vi "Versioned Load.vi"(10 "path":path) -> (0 "Reversals":T10, 1 "Trajectory Data":T1, 2 "Zero V":bool, 3 "Commands out":cluster{"Time (s)":dbl, T8, bool}[](array[cluster]), 4 "Fields":T7 {"Overrides"."Angle Override" step=5.0; "Overrides"."Velocity Override" step=5.0; "Overrides"."Angular Override" step=5.0; "Angular Limits"."Jerk (deg/s^3)" min=0.0 step=1.0; "Angular Limits"."Accel (deg/s^2)" min=0.0; "Angular Limits"."Velocity (deg/s)" min=0.0}, 5 "Points out":cluster{"x":dbl, "y":dbl, "th":dbl}[](array[cluster]), 6 "Trajectory Meta":cluster{"Drive Type":T3, "Path Type":T4}, 7 "Overall":cluster{"Time (s)":dbl, "Distance (ft)":dbl})   [LabVIEW 2025]
uses:
  Types/Single Cmd Info.ctl
  <vilib>/picture/picture.llb/imagedata.ctl
  Types/Overrides.ctl
  Types/Angluar Limits.ctl
  Types/Drive Type.ctl
  Types/Path Type.ctl
  Types/Trajectory Data.ctl
  Types/Segment Type.ctl
  Types/Availible Command systems for auto.ctl
  Types/Limits.ctl
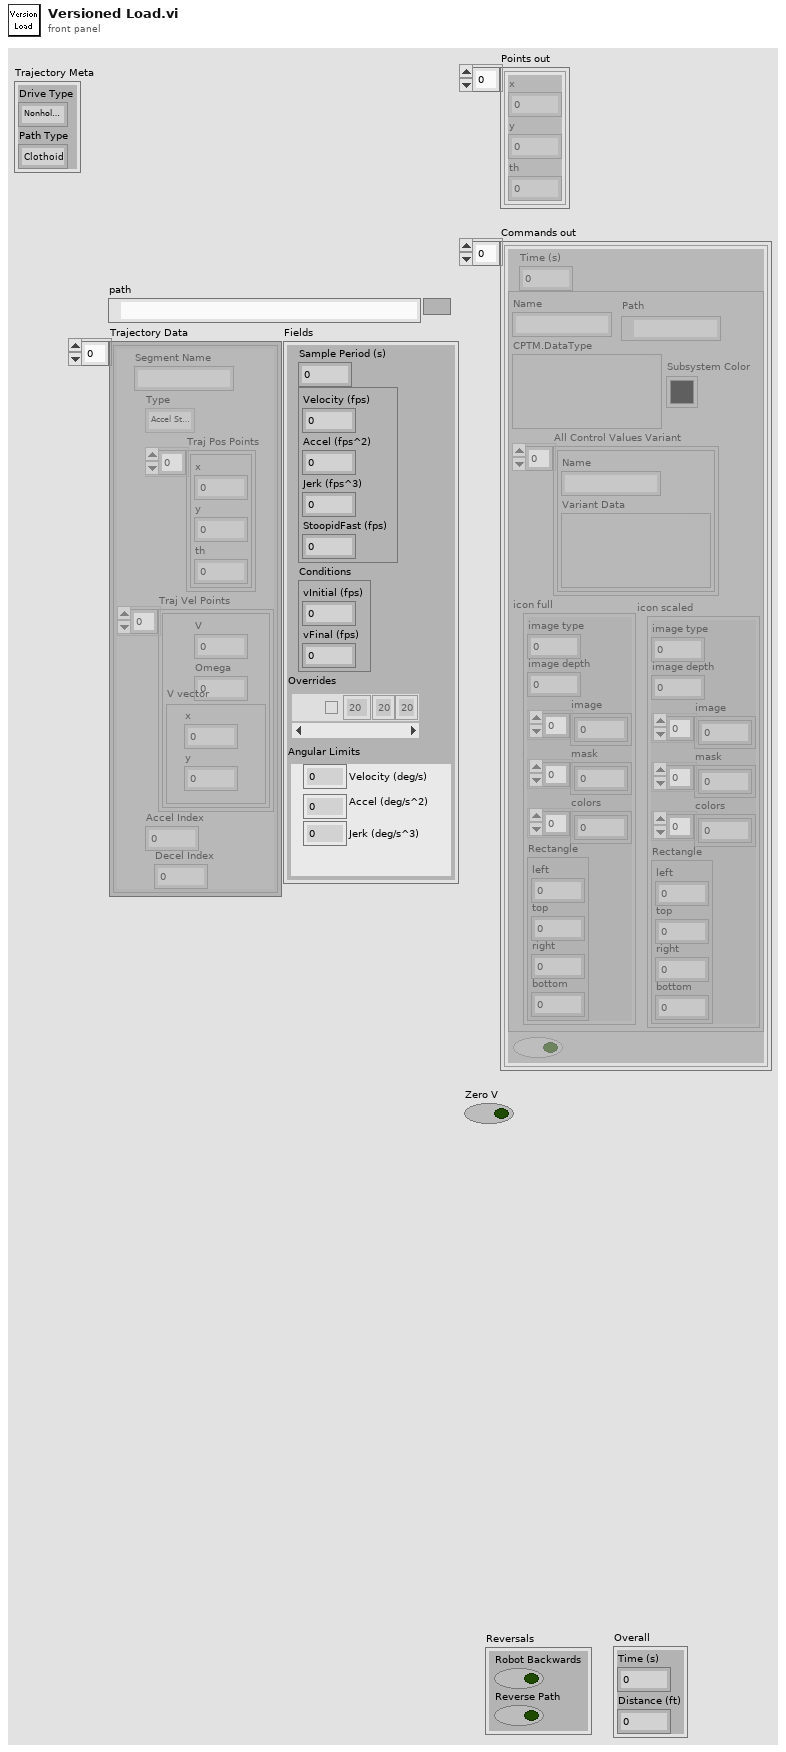
[diagram p1: front panel]
types:
  T1 = typedef "Trajectory Data.ctl" = cluster{"Segment Name":string, "Type":T2, "Traj Pos Points":cluster{"x":dbl, "y":dbl, "th":dbl}[], "Traj Vel Points":cluster{"V":dbl, "Omega":dbl, "V vector":cluster{"y":dbl, "x":dbl}}[], "Accel Index":i32, "Decel Index":i32}[]
  T2 = typedef "Segment Type.ctl" = enum16{"Accel Straight", "Const Straight", "Blend", "Circle", "Bezier"}
  T3 = typedef "Drive Type.ctl" = enum16{"Nonholonomic", "Holonomic"}
  T4 = typedef "Path Type.ctl" = enum16{"Clothoid", "Bezier"}
  T5 = typedef "Overrides.ctl" = cluster{"Count":string, "Angular Override":dbl, "Enabled?":bool, "Velocity Override":dbl, "Angle Override":dbl}[]
  T6 = typedef "Angluar Limits.ctl" = cluster{"Velocity (deg/s)":dbl, "Accel (deg/s^2)":dbl, "Jerk (deg/s^3)":dbl}
  T7 = cluster{"Sample Period (s)":dbl, cluster{"Velocity (fps)":dbl, "Accel (fps^2)":dbl, "Jerk (fps^3)":dbl, "StoopidFast (fps)":dbl}, "Conditions":cluster{"vInitial (fps)":dbl, "vFinal (fps)":dbl}, "Overrides":T5, "Angular Limits":T6}
  T8 = typedef "Single Cmd Info.ctl" = cluster{"Name":string, "CPTM.DataType":variant, "All Control Values Variant":cluster{"Name":string, "Variant Data":variant}[], "icon full":T9, "icon scaled":T9, "Path":path, "Subsystem Color":u32}
  T9 = typedef "imagedata.ctl" = cluster{"image type":i32, "image depth":i32, "image":u8[], "mask":u8[], "colors":u32[], "Rectangle":cluster{"left":i16, "top":i16, "right":i16, "bottom":i16}}
  T10 = cluster{"Robot Backwards":bool, "Reverse Path":bool}
  T11 = cluster{"Segment Name":string, "Type":T2, "Traj Pos Points":cluster{"x":dbl, "y":dbl, "th":dbl}[], "Traj Vel Points":cluster{"V":dbl, "Omega":dbl}[], "Accel Index":i32, "Decel Index":i32}[]
  T12 = cluster{"Sample Period (s)":dbl, "Limits 2":cluster{"Velocity (fps)":dbl, "Acceleration (fps^2)":dbl, "Jerk (fps^3)":dbl}, "Conditions":cluster{"vInitial (fps)":dbl, "vFinal (fps)":dbl}, " Acceleration Overrides":cluster{"Angular \nAccelerations":dbl[], "Accel Override Bools":bool[]}}
  T13 = cluster{"Velocity":dbl, "Sample Time":dbl, "Accel":dbl}
  T14 = cluster{"Sample Period (s)":dbl, "Limits":cluster{"Velocity (fps)":dbl, "Acceleration (fps^2)":dbl, "Jerk (fps^3)":dbl}, "Conditions":cluster{"vInitial (fps)":dbl, "vFinal (fps)":dbl}}
  T15 = cluster{"Sample Period (s)":dbl, "Limits":cluster{"Velocity (fps)":dbl, "Acceleration (fps^2)":dbl, "Jerk (fps^3)":dbl}, "Conditions":cluster{"vInitial (fps)":dbl, "vFinal (fps)":dbl}, "Min Rads":dbl[]}
  T16 = typedef "Availible Command systems for auto.ctl" = u16
  T17 = cluster{"Time into Path":dbl, "System":T16, "Item Selected?":bool, "System Selection":T16}[]
  T18 = cluster{"Sample Period (s)":dbl, "Limits 2":cluster{"Velocity (fps)":dbl, "Acceleration (fps^2)":dbl, "Jerk (fps^3)":dbl, "Stoopid Fast":dbl}, "Conditions":cluster{"vInitial (fps)":dbl, "vFinal (fps)":dbl}, " Acceleration Overrides":cluster{"Angular \nAccelerations":dbl[], "Accel Override Bools":bool[]}}
  T19 = cluster{"Sample Period (s)":dbl, "Limits":cluster{"Velocity (fps)":dbl, "Accel (fps^2)":dbl, "Turn Accel (fps^2)":dbl, "Jerk (fps^3)":dbl}, "Conditions":cluster{"vInitial (fps)":dbl, "vFinal (fps)":dbl}, cluster{dbl[], bool[]}}
  T20 = cluster{"Reverse Path":bool, "Robot Backwards":bool}
  T21 = typedef "Limits.ctl" = cluster{"Velocity (fps)":dbl, "Accel (fps^2)":dbl, "Jerk (fps^3)":dbl, "StoopidFast (fps)":dbl}
  T22 = cluster{"Sample Period (s)":dbl, "Limits":T21, "Conditions":cluster{"vInitial (fps)":dbl, "vFinal (fps)":dbl}, "Overrides":T5, "Angular Limits":T6}
  T23 = cluster{"Velocity":dbl, "Accel":dbl, "Accel":dbl, "Velocity":dbl}
  T24 = cluster{"Velocity (fps)":dbl, "Acceleration (fps^2)":dbl, "Jerk (fps^3)":dbl}
  T25 = cluster{"vInitial (fps)":dbl, "vFinal (fps)":dbl}
  T26 = cluster{"Velocity (fps)":dbl, "Acceleration (fps^2)":dbl, "Jerk (fps^3)":dbl, "Velocity (fps)":dbl}
  T27 = cluster{string, "Angular Multiplier":dbl, bool, "Velocity (fps)":dbl, "Velocity (fps)":dbl}
  T28 = cluster{"Angular \nAccelerations":dbl[], "Accel Override Bools":bool[]}
  T29 = cluster{"Velocity (fps)":dbl, "Acceleration (fps^2)":dbl, "Jerk (fps^3)":dbl, "Stoopid Fast":dbl}
  T30 = cluster{"Velocity (fps)":dbl, "Accel (fps^2)":dbl, "Turn Accel (fps^2)":dbl, "Jerk (fps^3)":dbl}
  T31 = cluster{"Velocity (fps)":dbl, "Accel (fps^2)":dbl, "Jerk (fps^3)":dbl, "StoopidFast (fps)":dbl}
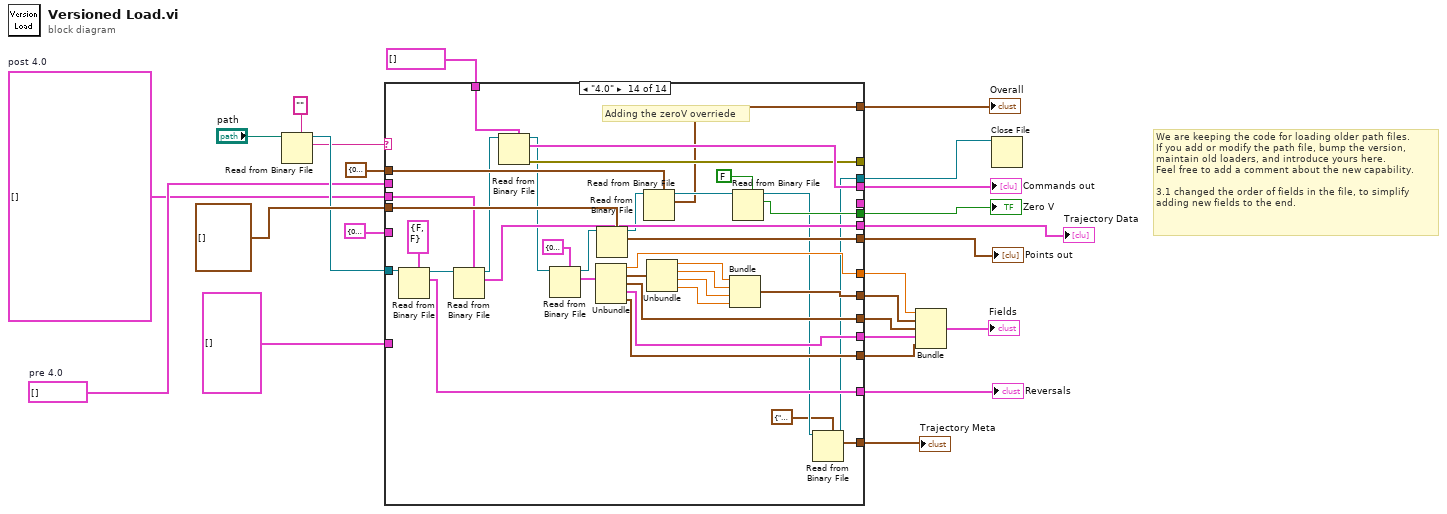
[diagram p0: block diagram]
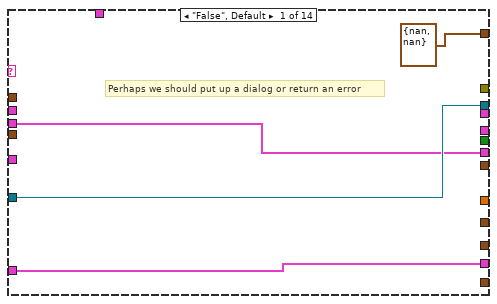
[diagram p2: hidden frame]
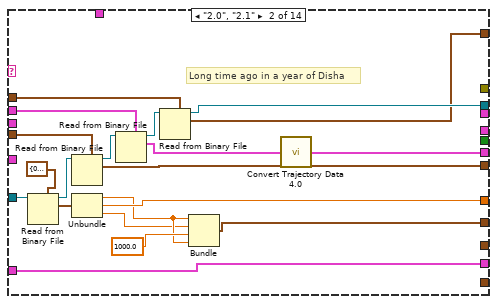
[diagram p3: hidden frame]
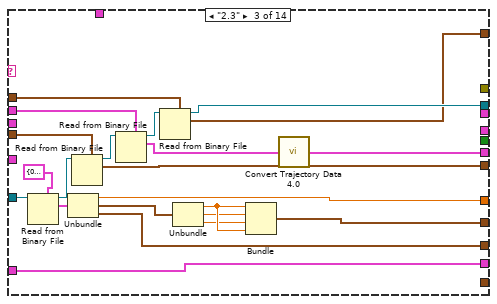
[diagram p4: hidden frame]
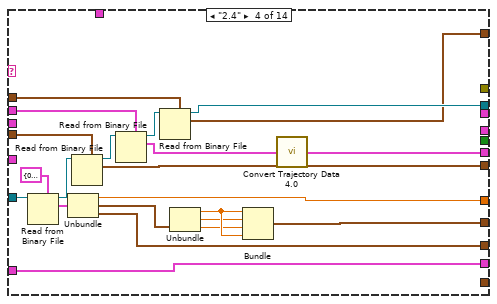
[diagram p5: hidden frame]
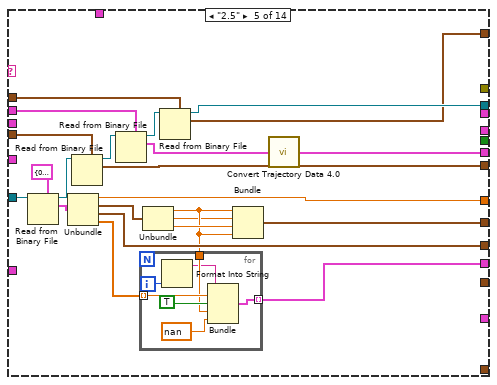
[diagram p6: hidden frame]
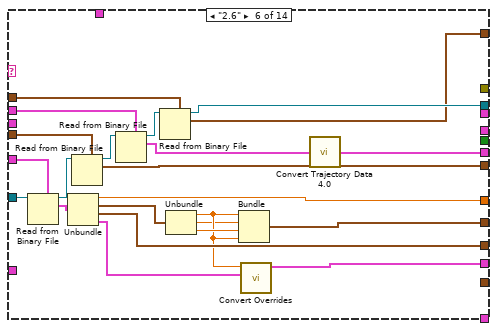
[diagram p7: hidden frame]
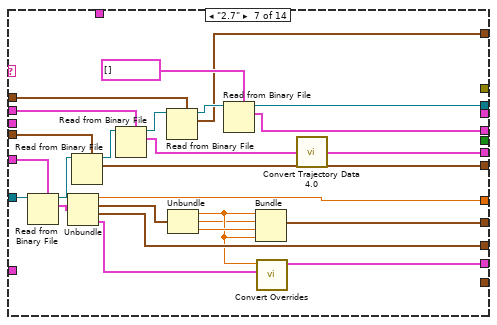
[diagram p8: hidden frame]
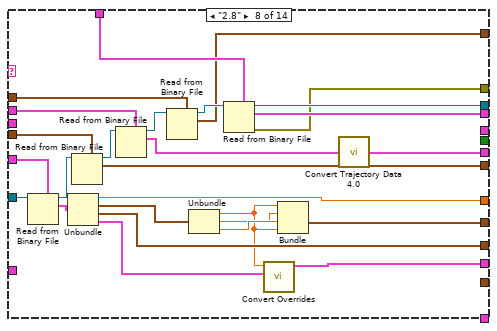
[diagram p9: hidden frame]
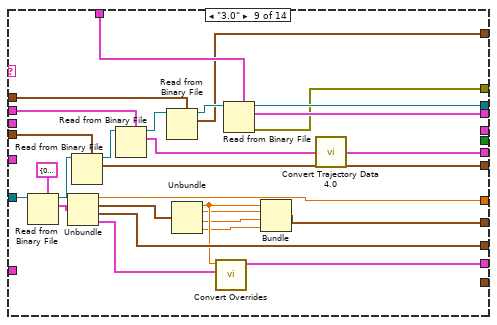
[diagram p10: hidden frame]
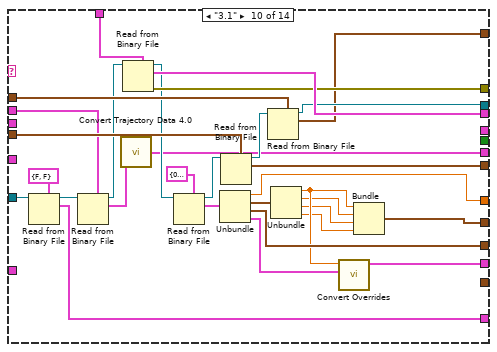
[diagram p11: hidden frame]
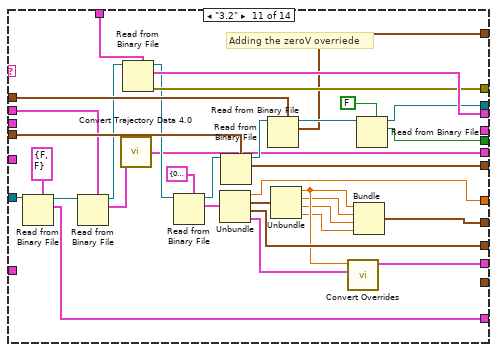
[diagram p12: hidden frame]
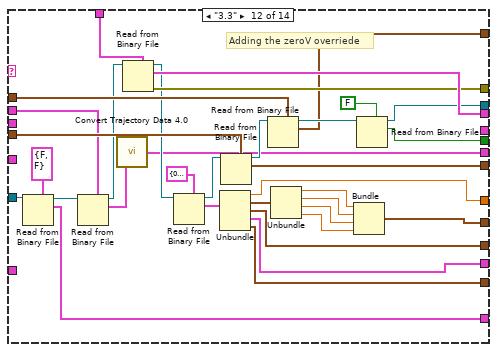
[diagram p13: hidden frame]
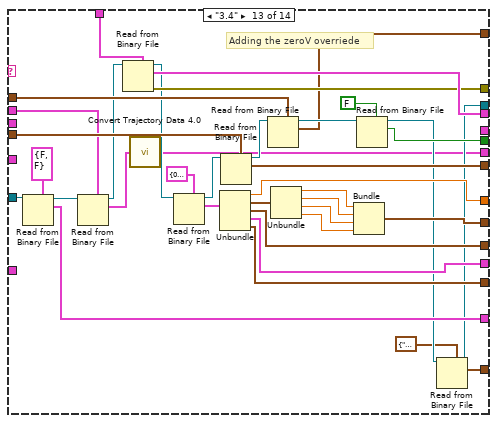
[diagram p14: hidden frame]
diagram:
  w3 = T11 []  # pre 4.0
  w2 = T1 []  # post 4.0
  # "We are keeping the code for loading older path files.\nIf you add or modify the path file, bump the version,\nmaintain old loaders, and introduce yours here.\nFeel free to add a comment about the new capability.\n\n3.1 changed the order of fields in the file, to simplify\nadding new fields to the end."
  n1 = Read from Binary File(5:"" ("String"), 11:"path") -> (2:w9:string, 3:w10:refnum<file>)  [unwired: 4 in, 2 out]
  n2 = case shown="\"4.0\"" w9 {
    tunnel: w10 -> [w29 w48 w70 w92 w115 w145 w171 w198 w226 w247 w281 w315 w352 w389]
    tunnel: cluster{"x":dbl, "y":dbl, "th":dbl}[] [] ("Points in") -> [_ w46 w68 w90 w113 w143 w169 w196 w224 w256 w290 w324 w361 w397]
    tunnel: [_ w45 w67 w89 w112 w142 w168 w195 w223 w255 w289 w323 w360 w396] -> w15
    tunnel: w3 -> [_ w44 w66 w88 w111 w141 w167 w194 w222 w254 w288 w322 w359 _]
    tunnel: cluster{"Time (s)":dbl, "Distance (ft)":dbl} {"Time (s)"=0.0, "Distance (ft)"=0.0} ("Cluster 4") -> [_ w42 w64 w86 w109 w139 w165 w192 w220 w253 w287 w321 w358 w395]
    tunnel: [w29 w40 w62 w84 w107 w137 w159 w186 w214 w243 w263 w300 w329 w366] -> w12
    tunnel: [_ w38 w61 w83 w106 w136 w163 w190 w218 w230 w265 w302 w339 w376] -> w22
    tunnel: [_ w34 w55 w76 w100 w131 w153 w181 w202 w235 w270 w307 w344 w381] -> w23
    tunnel: [_ _ w60 w82 w105 w135 w162 w189 w217 w252 w286 w320 w357 w394] -> w24
    tunnel: [w28 w33 w54 w75 w99 w129 w150 w178 w208 w239 w274 w295 w333 w370] -> w25
    tunnel: [w26 w30 w50 w72 w94 w124 w147 w173 w200 w228 w259 w293 w327 w393] -> w1
    tunnel: [_ _ _ _ _ _ w158 _ _ _ _ _ _ _] -> _
    tunnel: cluster{"Time (s)":dbl, T8, bool}[] [] ("Commands in") -> [_ _ _ _ _ _ _ w185 w213 w250 w284 w318 w355 w392]
    tunnel: [_ _ _ _ _ _ _ w184 w212 w249 w283 w317 w354 w391] -> w17
    tunnel: [_ _ _ _ _ _ _ w183 w211 w248 w282 w316 w353 w390] -> _
    tunnel: T12 {"Sample Period (s)"=0.0, "Limits 2"={"Velocity (fps)"=0.0, "Acceleration (fps^2)"=0.0, "Jerk (fps^3)"=0.0}, "Conditions"={"vInitial (fps)"=0.0, "vFinal (fps)"=0.0}, " Acceleration Overrides"={"Angular \nAccelerations"=[], "Accel Override Bools"=[]}} ("Cluster") -> [_ _ _ _ _ w133 w156 w179 _ _ _ _ _ _]
    tunnel: [_ _ _ _ _ _ _ _ _ w238 w273 w309 w346 w383] -> w19
    tunnel: T5 [] ("Overrides") -> [w28 w33 w54 w75 _ _ _ _ _ _ _ _ _ _]
    tunnel: [_ _ _ _ _ _ _ _ _ _ w261 w298 w336 w373] -> w20
    tunnel: [cluster{"Time (s)":dbl, "Distance (ft)":dbl} {"Time (s)"=nan, "Distance (ft)"=nan} ("Cluster 4") w31 w51 w73 w95 w125 w148 w174 w201 w229 w260 w297 w335 w372] -> w7
    tunnel: [_ _ _ _ _ _ _ _ _ _ _ w294 w332 w369] -> w5
    tunnel: [_ _ _ _ _ _ _ _ _ _ _ _ w328 w365] -> w4
    tunnel: w2 -> [w26 _ _ _ _ _ _ _ _ _ _ _ _ w364]
    frame "False", Default {
      # "Perhaps we should put up a dialog or return an error"
    }
    frame "2.0", "2.1" {
      # "Long time ago in a year of Disha"
      n3 = Read from Binary File(5:T13 {"Velocity"=0.0, "Sample Time"=0.0, "Accel"=0.0}, 11:w48) -> (2:w49:T13, 3:w47:refnum<file>)  [unwired: 4 in, 2 out]
      n4 = Read from Binary File(5:w46, 11:w47) -> (2:w45:cluster{"x":dbl, "y":dbl, "th":dbl}[], 3:w43:refnum<file>)  [unwired: 4 in, 2 out]
      n5 = Unbundle(w49) -> ("Velocity"=w35:dbl, "Sample Time"=w38:dbl, "Accel"=w32:dbl)
      n6 = Read from Binary File(5:w44, 11:w43) -> (2:w36:T11, 3:w41:refnum<file>)  [unwired: 4 in, 2 out]
      n7 = Read from Binary File(5:w42, 11:w41) -> (2:w31:cluster{"Time (s)":dbl, "Distance (ft)":dbl}, 3:w40:refnum<file>)  [unwired: 4 in, 2 out]
      n8 = Bundle("Velocity"=w35, "Accel"=w32, "Accel"=1000.0, "Velocity"=w35) -> (w34:T23)  [unwired: 1 in]
      n9 = call "Convert Trajectory Data 4.0.vi"("pre 4.0"=w36) -> ("post 4.0"=w30:T1)
    }
    frame "2.3" {
      n10 = Read from Binary File(5:T14 {"Sample Period (s)"=0.0, "Limits"={"Velocity (fps)"=0.0, "Acceleration (fps^2)"=0.0, "Jerk (fps^3)"=0.0}, "Conditions"={"vInitial (fps)"=0.0, "vFinal (fps)"=0.0}}, 11:w70) -> (2:w71:T14, 3:w69:refnum<file>)  [unwired: 4 in, 2 out]
      n11 = Unbundle(w71) -> ("Sample Period (s)"=w61:dbl, "Limits"=w52:T24, "Conditions"=w60:T25)
      n12 = Read from Binary File(5:w68, 11:w69) -> (2:w67:cluster{"x":dbl, "y":dbl, "th":dbl}[], 3:w65:refnum<file>)  [unwired: 4 in, 2 out]
      n13 = Read from Binary File(5:w66, 11:w65) -> (2:w58:T11, 3:w63:refnum<file>)  [unwired: 4 in, 2 out]
      n14 = Read from Binary File(5:w64, 11:w63) -> (2:w51:cluster{"Time (s)":dbl, "Distance (ft)":dbl}, 3:w62:refnum<file>)  [unwired: 4 in, 2 out]
      n15 = Unbundle(w52) -> ("Velocity (fps)"=w57:dbl, "Acceleration (fps^2)"=w53:dbl, "Jerk (fps^3)"=w56:dbl)
      n16 = Bundle("Velocity (fps)"=w57, "Acceleration (fps^2)"=w53, "Jerk (fps^3)"=w56, "Velocity (fps)"=w57) -> (w55:T26)  [unwired: 1 in]
      n17 = call "Convert Trajectory Data 4.0.vi"("pre 4.0"=w58) -> ("post 4.0"=w50:T1)
    }
    frame "2.4" {
      n18 = Read from Binary File(5:T14 {"Sample Period (s)"=0.0, "Limits"={"Velocity (fps)"=0.0, "Acceleration (fps^2)"=0.0, "Jerk (fps^3)"=0.0}, "Conditions"={"vInitial (fps)"=0.0, "vFinal (fps)"=0.0}}, 11:w92) -> (2:w93:T14, 3:w91:refnum<file>)  [unwired: 4 in, 2 out]
      n19 = Unbundle(w93) -> ("Sample Period (s)"=w83:dbl, "Limits"=w77:T24, "Conditions"=w82:T25)
      n20 = Read from Binary File(5:w90, 11:w91) -> (2:w89:cluster{"x":dbl, "y":dbl, "th":dbl}[], 3:w87:refnum<file>)  [unwired: 4 in, 2 out]
      n21 = Read from Binary File(5:w88, 11:w87) -> (2:w80:T11, 3:w85:refnum<file>)  [unwired: 4 in, 2 out]
      n22 = Read from Binary File(5:w86, 11:w85) -> (2:w73:cluster{"Time (s)":dbl, "Distance (ft)":dbl}, 3:w84:refnum<file>)  [unwired: 4 in, 2 out]
      n23 = Unbundle(w77) -> ("Velocity (fps)"=w79:dbl, "Acceleration (fps^2)"=w74:dbl, "Jerk (fps^3)"=w78:dbl)
      n24 = Bundle("Velocity (fps)"=w79, "Acceleration (fps^2)"=w74, "Jerk (fps^3)"=w78, "Velocity (fps)"=w79) -> (w76:T26)  [unwired: 1 in]
      n25 = call "Convert Trajectory Data 4.0.vi"("pre 4.0"=w80) -> ("post 4.0"=w72:T1)
    }
    frame "2.5" {
      n26 = Read from Binary File(5:T15 {"Sample Period (s)"=0.0, "Limits"={"Velocity (fps)"=0.0, "Acceleration (fps^2)"=0.0, "Jerk (fps^3)"=0.0}, "Conditions"={"vInitial (fps)"=0.0, "vFinal (fps)"=0.0}, "Min Rads"=[20.0, 20.0, 20.0, 20.0, 20.0]}, 11:w115) -> (2:w116:T15, 3:w114:refnum<file>)  [unwired: 4 in, 2 out]
      n27 = Unbundle(w116) -> ("Sample Period (s)"=w106:dbl, "Limits"=w101:T24, "Conditions"=w105:T25, "Min Rads"=w98:dbl[])
      n28 = Read from Binary File(5:w113, 11:w114) -> (2:w112:cluster{"x":dbl, "y":dbl, "th":dbl}[], 3:w110:refnum<file>)  [unwired: 4 in, 2 out]
      n29 = Read from Binary File(5:w111, 11:w110) -> (2:w103:T11, 3:w108:refnum<file>)  [unwired: 4 in, 2 out]
      n30 = Unbundle(w101) -> ("Velocity (fps)"=w97:dbl, "Acceleration (fps^2)"=w96:dbl, "Jerk (fps^3)"=w102:dbl)
      n31 = for {
        tunnel: [w122] -> w99 mode=indexing
        tunnel: w98 -> [w121] mode=indexing
        tunnel: w97 -> [w120]
        i -> [w119]
        n32 = Format Into String(w119) -> (resulting string=w118:string)  [unwired: 3 in, 1 out]
        n33 = Bundle(w118, "Angular Multiplier"=w121, TRUE, "Velocity (fps)"=w120, "Velocity (fps)"=nan) -> (w122:T27)  [unwired: 1 in]
      }
      n34 = Read from Binary File(5:w109, 11:w108) -> (2:w95:cluster{"Time (s)":dbl, "Distance (ft)":dbl}, 3:w107:refnum<file>)  [unwired: 4 in, 2 out]
      n35 = Bundle("Velocity (fps)"=w97, "Acceleration (fps^2)"=w96, "Jerk (fps^3)"=w102, "Velocity (fps)"=w97) -> (w100:T26)  [unwired: 1 in]
      n36 = call "Convert Trajectory Data 4.0.vi"("pre 4.0"=w103) -> ("post 4.0"=w94:T1)
    }
    frame "2.6" {
      n37 = Read from Binary File(5:w133, 11:w145) -> (2:w146:T12, 3:w144:refnum<file>)  [unwired: 4 in, 2 out]
      n38 = Unbundle(w146) -> ("Sample Period (s)"=w136:dbl, "Limits 2"=w130:T24, "Conditions"=w135:T25, "Acceleration Overrides"=w127:T28)
      n39 = Read from Binary File(5:w143, 11:w144) -> (2:w142:cluster{"x":dbl, "y":dbl, "th":dbl}[], 3:w140:refnum<file>)  [unwired: 4 in, 2 out]
      n40 = Read from Binary File(5:w141, 11:w140) -> (2:w134:T11, 3:w138:refnum<file>)  [unwired: 4 in, 2 out]
      n41 = Read from Binary File(5:w139, 11:w138) -> (2:w125:cluster{"Time (s)":dbl, "Distance (ft)":dbl}, 3:w137:refnum<file>)  [unwired: 4 in, 2 out]
      n42 = Unbundle(w130) -> ("Velocity (fps)"=w128:dbl, "Acceleration (fps^2)"=w126:dbl, "Jerk (fps^3)"=w132:dbl)
      n43 = Bundle("Velocity (fps)"=w128, "Acceleration (fps^2)"=w126, "Jerk (fps^3)"=w132, "Velocity (fps)"=w128) -> (w131:T26)  [unwired: 1 in]
      n44 = call "Convert Overrides.vi"("Cluster"=w127, "Velocity (fps)"=w128) -> ("Overrides"=w129:T5)  [unwired: 9 in]
      n45 = call "Convert Trajectory Data 4.0.vi"("pre 4.0"=w134) -> ("post 4.0"=w124:T1)
    }
    frame "2.7" {
      n46 = Read from Binary File(5:w156, 11:w171) -> (2:w172:T12, 3:w170:refnum<file>)  [unwired: 4 in, 2 out]
      n47 = Unbundle(w172) -> ("Sample Period (s)"=w163:dbl, "Limits 2"=w154:T24, "Conditions"=w162:T25, "Acceleration Overrides"=w151:T28)
      n48 = Read from Binary File(5:w169, 11:w170) -> (2:w168:cluster{"x":dbl, "y":dbl, "th":dbl}[], 3:w166:refnum<file>)  [unwired: 4 in, 2 out]
      n49 = Read from Binary File(5:w167, 11:w166) -> (2:w161:T11, 3:w164:refnum<file>)  [unwired: 4 in, 2 out]
      n50 = Read from Binary File(5:w165, 11:w164) -> (2:w148:cluster{"Time (s)":dbl, "Distance (ft)":dbl}, 3:w160:refnum<file>)  [unwired: 4 in, 2 out]
      n51 = Unbundle(w154) -> ("Velocity (fps)"=w152:dbl, "Acceleration (fps^2)"=w149:dbl, "Jerk (fps^3)"=w155:dbl)
      n52 = Read from Binary File(5:T17 [] ("Commands"), 11:w160) -> (2:w158:T17, 3:w159:refnum<file>)  [unwired: 4 in, 2 out]
      n53 = Bundle("Velocity (fps)"=w152, "Acceleration (fps^2)"=w149, "Jerk (fps^3)"=w155, "Velocity (fps)"=w152) -> (w153:T26)  [unwired: 1 in]
      n54 = call "Convert Overrides.vi"("Cluster"=w151, "Velocity (fps)"=w152) -> ("Overrides"=w150:T5)  [unwired: 9 in]
      n55 = call "Convert Trajectory Data 4.0.vi"("pre 4.0"=w161) -> ("post 4.0"=w147:T1)
    }
    frame "2.8" {
      n56 = Read from Binary File(5:w179, 11:w198) -> (2:w199:T12, 3:w197:refnum<file>)  [unwired: 4 in, 2 out]
      n57 = Unbundle(w199) -> ("Sample Period (s)"=w190:dbl, "Limits 2"=w182:T24, "Conditions"=w189:T25, "Acceleration Overrides"=w176:T28)
      n58 = Read from Binary File(5:w196, 11:w197) -> (2:w195:cluster{"x":dbl, "y":dbl, "th":dbl}[], 3:w193:refnum<file>)  [unwired: 4 in, 2 out]
      n59 = Read from Binary File(5:w194, 11:w193) -> (2:w188:T11, 3:w191:refnum<file>)  [unwired: 4 in, 2 out]
      n60 = Read from Binary File(5:w192, 11:w191) -> (2:w174:cluster{"Time (s)":dbl, "Distance (ft)":dbl}, 3:w187:refnum<file>)  [unwired: 4 in, 2 out]
      n61 = Unbundle(w182) -> ("Velocity (fps)"=w177:dbl, "Acceleration (fps^2)"=w175:dbl, "Jerk (fps^3)"=w180:dbl)
      n62 = Read from Binary File(5:w185, 11:w187) -> (0:w183:errorcluster, 2:w184:cluster{"Time (s)":dbl, T8, bool}[], 3:w186:refnum<file>)  [unwired: 4 in, 1 out]
      n63 = call "Convert Overrides.vi"("Cluster"=w176, "Velocity (fps)"=w177) -> ("Overrides"=w178:T5)  [unwired: 9 in]
      n64 = Bundle("Velocity (fps)"=w177, "Acceleration (fps^2)"=w175, "Jerk (fps^3)"=w180, "Velocity (fps)"=w177) -> (w181:T26)  [unwired: 1 in]
      n65 = call "Convert Trajectory Data 4.0.vi"("pre 4.0"=w188) -> ("post 4.0"=w173:T1)
    }
    frame "3.0" {
      n66 = Read from Binary File(5:T18 {"Sample Period (s)"=0.0, "Limits 2"={"Velocity (fps)"=0.0, "Acceleration (fps^2)"=0.0, "Jerk (fps^3)"=0.0, "Stoopid Fast"=0.0}, "Conditions"={"vInitial (fps)"=0.0, "vFinal (fps)"=0.0}, " Acceleration Overrides"={"Angular \nAccelerations"=[], "Accel Override Bools"=[]}} ("Cluster"), 11:w226) -> (2:w227:T18, 3:w225:refnum<file>)  [unwired: 4 in, 2 out]
      n67 = Unbundle(w227) -> ("Sample Period (s)"=w218:dbl, "Limits 2"=w203:T29, "Conditions"=w217:T25, "Acceleration Overrides"=w209:T28)
      n68 = Read from Binary File(5:w224, 11:w225) -> (2:w223:cluster{"x":dbl, "y":dbl, "th":dbl}[], 3:w221:refnum<file>)  [unwired: 4 in, 2 out]
      n69 = Read from Binary File(5:w222, 11:w221) -> (2:w216:T11, 3:w219:refnum<file>)  [unwired: 4 in, 2 out]
      n70 = Read from Binary File(5:w220, 11:w219) -> (2:w201:cluster{"Time (s)":dbl, "Distance (ft)":dbl}, 3:w215:refnum<file>)  [unwired: 4 in, 2 out]
      n71 = Unbundle(w203) -> ("Velocity (fps)"=w207:dbl, "Acceleration (fps^2)"=w206:dbl, "Jerk (fps^3)"=w205:dbl, "Stoopid Fast"=w204:dbl)
      n72 = call "Convert Overrides.vi"("Cluster"=w209, "Velocity (fps)"=w207) -> ("Overrides"=w208:T5)  [unwired: 9 in]
      n73 = Read from Binary File(5:w213, 11:w215) -> (0:w211:errorcluster, 2:w212:cluster{"Time (s)":dbl, T8, bool}[], 3:w214:refnum<file>)  [unwired: 4 in, 1 out]
      n74 = Bundle("Velocity (fps)"=w207, "Acceleration (fps^2)"=w206, "Jerk (fps^3)"=w205, "Stoopid Fast"=w204) -> (w202:T29)  [unwired: 1 in]
      n75 = call "Convert Trajectory Data 4.0.vi"("pre 4.0"=w216) -> ("post 4.0"=w200:T1)
    }
    frame "3.1" {
      n76 = Read from Binary File(5:T20 {"Reverse Path"=FALSE, "Robot Backwards"=FALSE} ("Cluster"), 11:w247) -> (2:w238:T20, 3:w244:refnum<file>)  [unwired: 4 in, 2 out]
      n77 = Read from Binary File(5:w254, 11:w244) -> (2:w251:T11, 3:w242:refnum<file>)  [unwired: 4 in, 2 out]
      n78 = call "Convert Trajectory Data 4.0.vi"("pre 4.0"=w251) -> ("post 4.0"=w228:T1)
      n79 = Read from Binary File(5:w250, 11:w242) -> (0:w248:errorcluster, 2:w249:cluster{"Time (s)":dbl, T8, bool}[], 3:w241:refnum<file>)  [unwired: 4 in, 1 out]
      n80 = Read from Binary File(5:T19 {"Sample Period (s)"=0.0, "Limits"={"Velocity (fps)"=0.0, "Accel (fps^2)"=0.0, "Turn Accel (fps^2)"=15.0, "Jerk (fps^3)"=0.0}, "Conditions"={"vInitial (fps)"=0.0, "vFinal (fps)"=0.0}, {[], []}} ("Cluster 2"), 11:w241) -> (2:w258:T19, 3:w257:refnum<file>)  [unwired: 4 in, 2 out]
      n81 = Unbundle(w258) -> ("Sample Period (s)"=w230:dbl, "Limits"=w237:T30, "Conditions"=w252:T25, w240:cluster{dbl[], bool[]})
      n82 = Read from Binary File(5:w256, 11:w257) -> (2:w255:cluster{"x":dbl, "y":dbl, "th":dbl}[], 3:w245:refnum<file>)  [unwired: 4 in, 2 out]
      n83 = Read from Binary File(5:w253, 11:w245) -> (2:w229:cluster{"Time (s)":dbl, "Distance (ft)":dbl}, 3:w243:refnum<file>)  [unwired: 4 in, 2 out]
      n84 = Unbundle(w237) -> ("Velocity (fps)"=w234:dbl, "Accel (fps^2)"=w233:dbl, "Turn Accel (fps^2)"=w232:dbl, "Jerk (fps^3)"=w231:dbl)
      n85 = call "Convert Overrides.vi"("Cluster"=w240, "Velocity (fps)"=w234) -> ("Overrides"=w239:T5)  [unwired: 9 in]
      n86 = Bundle("Velocity (fps)"=w234, "Accel (fps^2)"=w233, "Turn Accel (fps^2)"=w232, "Jerk (fps^3)"=w231) -> (w235:T30)  [unwired: 1 in]
    }
    frame "3.2" {
      # "Adding the zeroV overriede"
      n87 = Read from Binary File(5:T10 {"Robot Backwards"=FALSE, "Reverse Path"=FALSE} ("Cluster"), 11:w281) -> (2:w273:T10, 3:w278:refnum<file>)  [unwired: 4 in, 2 out]
      n88 = Read from Binary File(5:w288, 11:w278) -> (2:w285:T11, 3:w277:refnum<file>)  [unwired: 4 in, 2 out]
      n89 = call "Convert Trajectory Data 4.0.vi"("pre 4.0"=w285) -> ("post 4.0"=w259:T1)
      n90 = Read from Binary File(5:w284, 11:w277) -> (0:w282:errorcluster, 2:w283:cluster{"Time (s)":dbl, T8, bool}[], 3:w276:refnum<file>)  [unwired: 4 in, 1 out]
      n91 = Read from Binary File(5:T19 {"Sample Period (s)"=0.0, "Limits"={"Velocity (fps)"=0.0, "Accel (fps^2)"=0.0, "Turn Accel (fps^2)"=15.0, "Jerk (fps^3)"=0.0}, "Conditions"={"vInitial (fps)"=0.0, "vFinal (fps)"=0.0}, {[], []}} ("Cluster 2"), 11:w276) -> (2:w292:T19, 3:w291:refnum<file>)  [unwired: 4 in, 2 out]
      n92 = Unbundle(w292) -> ("Sample Period (s)"=w265:dbl, "Limits"=w272:T30, "Conditions"=w286:T25, w275:cluster{dbl[], bool[]})
      n93 = Read from Binary File(5:w290, 11:w291) -> (2:w289:cluster{"x":dbl, "y":dbl, "th":dbl}[], 3:w279:refnum<file>)  [unwired: 4 in, 2 out]
      n94 = Read from Binary File(5:w287, 11:w279) -> (2:w260:cluster{"Time (s)":dbl, "Distance (ft)":dbl}, 3:w264:refnum<file>)  [unwired: 4 in, 2 out]
      n95 = Unbundle(w272) -> ("Velocity (fps)"=w269:dbl, "Accel (fps^2)"=w268:dbl, "Turn Accel (fps^2)"=w267:dbl, "Jerk (fps^3)"=w266:dbl)
      n96 = call "Convert Overrides.vi"("Cluster"=w275, "Velocity (fps)"=w269) -> ("Overrides"=w274:T5)  [unwired: 9 in]
      n97 = Bundle("Velocity (fps)"=w269, "Accel (fps^2)"=w268, "Turn Accel (fps^2)"=w267, "Jerk (fps^3)"=w266) -> (w270:T30)  [unwired: 1 in]
      n98 = Read from Binary File(5:FALSE, 11:w264) -> (2:w261:bool, 3:w263:refnum<file>)  [unwired: 4 in, 2 out]
    }
    frame "3.3" {
      # "Adding the zeroV overriede"
      n99 = Read from Binary File(5:T10 {"Robot Backwards"=FALSE, "Reverse Path"=FALSE} ("Cluster"), 11:w315) -> (2:w309:T10, 3:w312:refnum<file>)  [unwired: 4 in, 2 out]
      n100 = Read from Binary File(5:w322, 11:w312) -> (2:w319:T11, 3:w311:refnum<file>)  [unwired: 4 in, 2 out]
      n101 = call "Convert Trajectory Data 4.0.vi"("pre 4.0"=w319) -> ("post 4.0"=w293:T1)
      n102 = Read from Binary File(5:w318, 11:w311) -> (0:w316:errorcluster, 2:w317:cluster{"Time (s)":dbl, T8, bool}[], 3:w310:refnum<file>)  [unwired: 4 in, 1 out]
      n103 = Read from Binary File(5:T22 {"Sample Period (s)"=0.0, "Limits"={"Velocity (fps)"=0.0, "Accel (fps^2)"=0.0, "Jerk (fps^3)"=0.0, "StoopidFast (fps)"=0.0}, "Conditions"={"vInitial (fps)"=0.0, "vFinal (fps)"=0.0}, "Overrides"=[], "Angular Limits"={"Velocity (deg/s)"=0.0, "Accel (deg/s^2)"=0.0, "Jerk (deg/s^3)"=0.0}} ("output cluster"), 11:w310) -> (2:w326:T22, 3:w325:refnum<file>)  [unwired: 4 in, 2 out]
      n104 = Unbundle(w326) -> ("Sample Period (s)"=w302:dbl, "Limits"=w308:T21, "Conditions"=w320:T25, "Overrides"=w295:T5, "Angular Limits"=w294:T6)
      n105 = Read from Binary File(5:w324, 11:w325) -> (2:w323:cluster{"x":dbl, "y":dbl, "th":dbl}[], 3:w313:refnum<file>)  [unwired: 4 in, 2 out]
      n106 = Read from Binary File(5:w321, 11:w313) -> (2:w297:cluster{"Time (s)":dbl, "Distance (ft)":dbl}, 3:w301:refnum<file>)  [unwired: 4 in, 2 out]
      n107 = Unbundle(w308) -> ("Velocity (fps)"=w306:dbl, "Accel (fps^2)"=w305:dbl, "Jerk (fps^3)"=w304:dbl, "StoopidFast (fps)"=w303:dbl)
      n108 = Bundle("Velocity (fps)"=w306, "Accel (fps^2)"=w305, "Jerk (fps^3)"=w304, "StoopidFast (fps)"=w303) -> (w307:T31)  [unwired: 1 in]
      n109 = Read from Binary File(5:FALSE, 11:w301) -> (2:w298:bool, 3:w300:refnum<file>)  [unwired: 4 in, 2 out]
    }
    frame "3.4" {
      # "Adding the zeroV overriede"
      n110 = Read from Binary File(5:T10 {"Robot Backwards"=FALSE, "Reverse Path"=FALSE} ("Cluster"), 11:w352) -> (2:w346:T10, 3:w349:refnum<file>)  [unwired: 4 in, 2 out]
      n111 = Read from Binary File(5:w359, 11:w349) -> (2:w356:T11, 3:w348:refnum<file>)  [unwired: 4 in, 2 out]
      n112 = Read from Binary File(5:w355, 11:w348) -> (0:w353:errorcluster, 2:w354:cluster{"Time (s)":dbl, T8, bool}[], 3:w347:refnum<file>)  [unwired: 4 in, 1 out]
      n113 = call "Convert Trajectory Data 4.0.vi"("pre 4.0"=w356) -> ("post 4.0"=w327:T1)
      n114 = Read from Binary File(5:T22 {"Sample Period (s)"=0.0, "Limits"={"Velocity (fps)"=0.0, "Accel (fps^2)"=0.0, "Jerk (fps^3)"=0.0, "StoopidFast (fps)"=0.0}, "Conditions"={"vInitial (fps)"=0.0, "vFinal (fps)"=0.0}, "Overrides"=[], "Angular Limits"={"Velocity (deg/s)"=0.0, "Accel (deg/s^2)"=0.0, "Jerk (deg/s^3)"=0.0}} ("output cluster"), 11:w347) -> (2:w363:T22, 3:w362:refnum<file>)  [unwired: 4 in, 2 out]
      n115 = Unbundle(w363) -> ("Sample Period (s)"=w339:dbl, "Limits"=w345:T21, "Conditions"=w357:T25, "Overrides"=w333:T5, "Angular Limits"=w332:T6)
      n116 = Read from Binary File(5:w361, 11:w362) -> (2:w360:cluster{"x":dbl, "y":dbl, "th":dbl}[], 3:w350:refnum<file>)  [unwired: 4 in, 2 out]
      n117 = Read from Binary File(5:w358, 11:w350) -> (2:w335:cluster{"Time (s)":dbl, "Distance (ft)":dbl}, 3:w338:refnum<file>)  [unwired: 4 in, 2 out]
      n118 = Unbundle(w345) -> ("Velocity (fps)"=w343:dbl, "Accel (fps^2)"=w342:dbl, "Jerk (fps^3)"=w341:dbl, "StoopidFast (fps)"=w340:dbl)
      n119 = Bundle("Velocity (fps)"=w343, "Accel (fps^2)"=w342, "Jerk (fps^3)"=w341, "StoopidFast (fps)"=w340) -> (w344:T31)  [unwired: 1 in]
      n120 = Read from Binary File(5:FALSE, 11:w338) -> (2:w336:bool, 3:w331:refnum<file>)  [unwired: 4 in, 2 out]
      n121 = Read from Binary File(5:cluster{"Drive Type":T3, "Path Type":T4} {"Drive Type"=enum."Nonholonomic", "Path Type"=enum."Clothoid"} ("Trajectory Meta"), 11:w331) -> (2:w328:cluster{"Drive Type":T3, "Path Type":T4}, 3:w329:refnum<file>)  [unwired: 4 in, 2 out]
    }
    frame "4.0" {
      # "Adding the zeroV overriede"
      n122 = Read from Binary File(5:T10 {"Robot Backwards"=FALSE, "Reverse Path"=FALSE} ("Cluster"), 11:w389) -> (2:w383:T10, 3:w386:refnum<file>)  [unwired: 4 in, 2 out]
      n123 = Read from Binary File(5:w364, 11:w386) -> (2:w393:T1, 3:w385:refnum<file>)  [unwired: 4 in, 2 out]
      n124 = Read from Binary File(5:w392, 11:w385) -> (0:w390:errorcluster, 2:w391:cluster{"Time (s)":dbl, T8, bool}[], 3:w384:refnum<file>)  [unwired: 4 in, 1 out]
      n125 = Read from Binary File(5:T22 {"Sample Period (s)"=0.0, "Limits"={"Velocity (fps)"=0.0, "Accel (fps^2)"=0.0, "Jerk (fps^3)"=0.0, "StoopidFast (fps)"=0.0}, "Conditions"={"vInitial (fps)"=0.0, "vFinal (fps)"=0.0}, "Overrides"=[], "Angular Limits"={"Velocity (deg/s)"=0.0, "Accel (deg/s^2)"=0.0, "Jerk (deg/s^3)"=0.0}} ("output cluster"), 11:w384) -> (2:w399:T22, 3:w398:refnum<file>)  [unwired: 4 in, 2 out]
      n126 = Unbundle(w399) -> ("Sample Period (s)"=w376:dbl, "Limits"=w382:T21, "Conditions"=w394:T25, "Overrides"=w370:T5, "Angular Limits"=w369:T6)
      n127 = Read from Binary File(5:w397, 11:w398) -> (2:w396:cluster{"x":dbl, "y":dbl, "th":dbl}[], 3:w387:refnum<file>)  [unwired: 4 in, 2 out]
      n128 = Read from Binary File(5:w395, 11:w387) -> (2:w372:cluster{"Time (s)":dbl, "Distance (ft)":dbl}, 3:w375:refnum<file>)  [unwired: 4 in, 2 out]
      n129 = Unbundle(w382) -> ("Velocity (fps)"=w380:dbl, "Accel (fps^2)"=w379:dbl, "Jerk (fps^3)"=w378:dbl, "StoopidFast (fps)"=w377:dbl)
      n130 = Bundle("Velocity (fps)"=w380, "Accel (fps^2)"=w379, "Jerk (fps^3)"=w378, "StoopidFast (fps)"=w377) -> (w381:T31)  [unwired: 1 in]
      n131 = Read from Binary File(5:FALSE, 11:w375) -> (2:w373:bool, 3:w368:refnum<file>)  [unwired: 4 in, 2 out]
      n132 = Read from Binary File(5:cluster{"Drive Type":T3, "Path Type":T4} {"Drive Type"=enum."Nonholonomic", "Path Type"=enum."Clothoid"} ("Trajectory Meta"), 11:w368) -> (2:w365:cluster{"Drive Type":T3, "Path Type":T4}, 3:w366:refnum<file>)  [unwired: 4 in, 2 out]
    }
  }
  "Zero V" <- w20
  "Reversals" <- w19
  "Commands out" <- w17
  "Points out" <- w15
  "Overall" <- w7
  "Trajectory Meta" <- w4
  "Trajectory Data" <- w1
  n133 = Bundle("Sample Period (s)"=w22, w23, "Conditions"=w24, "Overrides"=w25, "Angular Limits"=w5) -> (→"Fields":T7)  [unwired: 1 in]
  n134 = Close File(refnum=w12) -> ()  [unwired: 1 in, 2 out]
